vi "sedSpectrometer_logEvent_detailedState.vi"(8 "error in (no error)":errorcluster, 11 "logevent_detailedState_Ctl":T1) -> (0 "error out":errorcluster, 2 "function return":i32, 3 "logevent_detailedState_Ctl out":T1)   [LabVIEW 2016, in "SALLV_sedSpectrometer.lvlib"]
doc: "int sedSpectrometer_shm_logEvent_detailedStateLV(sedSpectrometer_logevent_detailedStateLV *logevent_detailedState_Ctl );"
uses:
  SALLV_sedSpectrometer.lvlib
  DataTypes/logevent_detailedState.ctl
  SALLV_sedSpectrometer.so
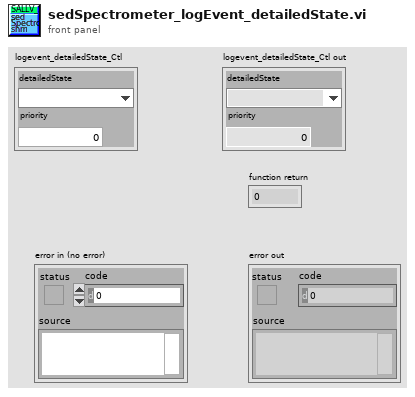
[diagram p1: front panel]
types:
  T1 = typedef "SALLV_sedSpectrometer.lvlib/logevent_detailedState.ctl" = cluster{"detailedState":enum32{"", "DisabledState", "EnabledState", "FaultState", "OfflineState", "StandbyState", "ImagingState", "NotImagingState"}, "priority":i32}
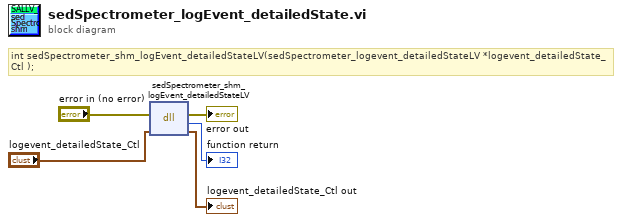
[diagram p0: block diagram]
diagram:
  # "int sedSpectrometer_shm_logEvent_detailedStateLV(sedSpectrometer_logevent_detailedStateLV *logevent_detailedState_Ctl );"
  n1 = dll-call lib="home/harini/tcs/ts_sedspectrometer/ts_sallv_sedspectrometer/SALLV_sedSpectrometer.*" fn="sedSpectrometer_shm_logEvent_detailedStateLV"(error in="error in (no error)", "logevent_detailedState_Ctl"="logevent_detailedState_Ctl") -> (error out=→"error out":errorcluster, →"function return":i32, "logevent_detailedState_Ctl"=→"logevent_detailedState_Ctl out":T1)  [unwired: 2 in, 1 out]
